vi "Close.vi"(8 "error in (no error)":errorcluster, 11 "State in":T1={"State"=enum."Idle", "Start Time"=timestamp(0 s since 1904-01-01), "Configuration"={"Cycle Period"=0.0, "PID 2 Parameters"={"Input Device"=enum."4-20mA", "Output Device"=enum."Default", "Setpoint"=0.0, "PID gains"={"proportional gain (Kc)"=0.0, "integral time (Ti, min)"=0.0, "derivative time (Td, min)"=100.0}, "output range"={"output low"=0.0, "output high"=1.0}}, "Manual Entry"=0.0, "Auto?"=TRUE, "4-20mA Input Settings"={"Input Channel "=0}, "4-20mA Out Settings"={"Output DAQ Task"=""}, "Input Channel Tag Name "=""}, "Current Time"=timestamp(0 s since 1904-01-01), "PID 1 Parameters"={"Setpoint"=0.0, "PID gains"={"proportional gain (Kc)"=1.0, "integral time (Ti, min)"=0.01, "derivative time (Td, min)"=0.0}}, "First Iteration"=FALSE, "Data"={"4-20mA Input"=0.0, "PID 2 Process Variable"=0.0, "PID 2 Output"=0.0, "4-20mA Output"=0.0}, "Process Name"="", "Pump On?"=enum."Off", "Input Error"=FALSE, "Output Error"=FALSE, "Log Started"=FALSE} {"Configuration"."PID 2 Parameters"."output range"."output low" format="%.2f"; "Configuration"."PID 2 Parameters"."output range"."output high" min=0.0 max=100.0 format="%.2f"; "Configuration"."PID 2 Parameters"."PID gains"."derivative time (Td, min)" format="%.3f"; "Configuration"."PID 2 Parameters"."PID gains"."integral time (Ti, min)" format="%.3f"; "Configuration"."PID 2 Parameters"."PID gains"."proportional gain (Kc)" format="%.3f"; "PID 1 Parameters"."PID gains"."derivative time (Td, min)" format="%.3f"; "PID 1 Parameters"."PID gains"."integral time (Ti, min)" format="%.3f"; "PID 1 Parameters"."PID gains"."proportional gain (Kc)" format="%.3f"}) -> (0 "error out":errorcluster, 3 "State out":T1={"State"=enum."Idle", "Start Time"=timestamp(0 s since 1904-01-01), "Configuration"={"Cycle Period"=0.0, "PID 2 Parameters"={"Input Device"=enum."4-20mA", "Output Device"=enum."Default", "Setpoint"=0.0, "PID gains"={"proportional gain (Kc)"=0.0, "integral time (Ti, min)"=0.0, "derivative time (Td, min)"=100.0}, "output range"={"output low"=0.0, "output high"=1.0}}, "Manual Entry"=0.0, "Auto?"=TRUE, "4-20mA Input Settings"={"Input Channel "=0}, "4-20mA Out Settings"={"Output DAQ Task"=""}, "Input Channel Tag Name "=""}, "Current Time"=timestamp(0 s since 1904-01-01), "PID 1 Parameters"={"Setpoint"=0.0, "PID gains"={"proportional gain (Kc)"=1.0, "integral time (Ti, min)"=0.01, "derivative time (Td, min)"=0.0}}, "First Iteration"=FALSE, "Data"={"4-20mA Input"=0.0, "PID 2 Process Variable"=0.0, "PID 2 Output"=0.0, "4-20mA Output"=0.0}, "Process Name"="", "Pump On?"=enum."Off", "Input Error"=FALSE, "Output Error"=FALSE, "Log Started"=FALSE} {"Configuration"."PID 2 Parameters"."output range"."output low" format="%.2f"; "Configuration"."PID 2 Parameters"."output range"."output high" min=0.0 max=100.0 format="%.2f"; "Configuration"."PID 2 Parameters"."PID gains"."derivative time (Td, min)" format="%.3f"; "Configuration"."PID 2 Parameters"."PID gains"."integral time (Ti, min)" format="%.3f"; "Configuration"."PID 2 Parameters"."PID gains"."proportional gain (Kc)" format="%.3f"; "PID 1 Parameters"."PID gains"."derivative time (Td, min)" format="%.3f"; "PID 1 Parameters"."PID gains"."integral time (Ti, min)" format="%.3f"; "PID 1 Parameters"."PID gains"."proportional gain (Kc)" format="%.3f"})   [LabVIEW 2018, in "4-20mA Module.lvlib" / "4-20mA Module Engine.lvlib"]
uses:
  4-20mA Module Engine.lvlib
  State Cluster.ctl
  State Enum.ctl
  Pressure Transmitter/Pressure Transmitter Device Settings.ctl
  Pressure Reg Module/Pressure Regulator Device Settings.ctl
  Measure Instrument/PID 1 Parameters Cluster.ctl
  Pressure Transmitter/Pressure Transmitter Library.lvlib
  Pressure Reg Module/Pressure Regulator Library.lvlib
panel:
  # "Instrument Settings"
  # "Instrument Settings"
  # "Instrument Settings"
  # "Instrument Settings"
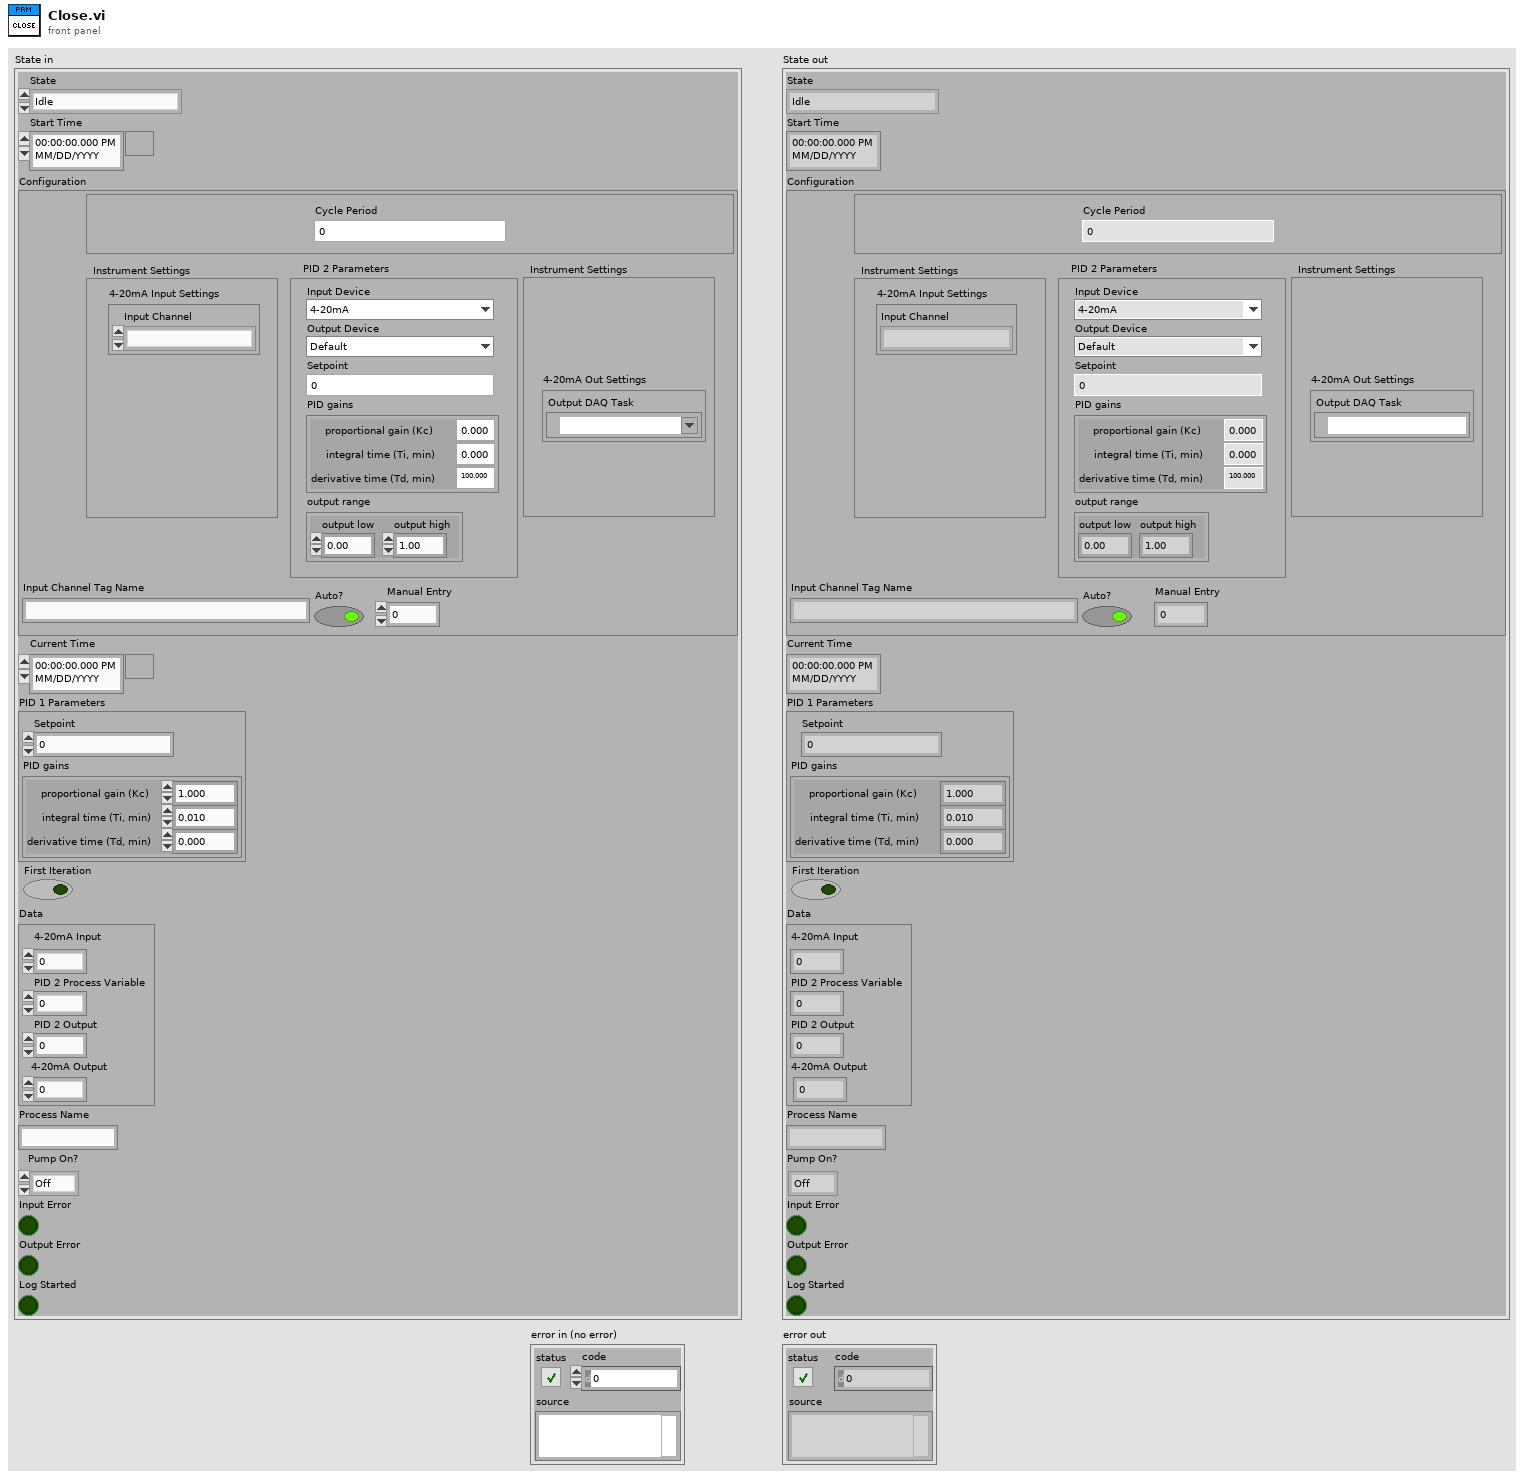
[diagram p1: front panel]
types:
  T1 = typedef "4-20mA Module.lvlib/4-20mA Module Engine.lvlib/State Cluster.ctl" = cluster{"State":T2, "Start Time":timestamp, "Configuration":cluster{"Cycle Period":dbl, "PID 2 Parameters":cluster{"Input Device":enum16{"Default", "4-20mA"}, "Output Device":enum16{"Default", "4-20mA"}, "Setpoint":dbl, "PID gains":cluster{"proportional gain (Kc)":dbl, "integral time (Ti, min)":dbl, "derivative time (Td, min)":dbl}, "output range":cluster{"output low":dbl, "output high":dbl}}, "Manual Entry":dbl, "Auto?":bool, "4-20mA Input Settings":T3, "4-20mA Out Settings":T4, "Input Channel Tag Name ":string}, "Current Time":timestamp, "PID 1 Parameters":T5, "First Iteration":bool, "Data":cluster{"4-20mA Input":dbl, "PID 2 Process Variable":dbl, "PID 2 Output":dbl, "4-20mA Output":dbl}, "Process Name":string, "Pump On?":enum16{"Off", "On", "Not Initialized"}, "Input Error":bool, "Output Error":bool, "Log Started":bool}
  T2 = typedef "4-20mA Module.lvlib/4-20mA Module Engine.lvlib/State Enum.ctl" = enum16{"Measuring", "Idle", "Paused"}
  T3 = typedef "Pressure Transmitter Library.lvlib/Pressure Transmitter Device Settings.ctl" = cluster{"Input Channel ":u16}
  T4 = typedef "Pressure Regulator Library.lvlib/Pressure Regulator Device Settings.ctl" = cluster{"Output DAQ Task":refnum<k21>}
  T5 = typedef "PID 1 Parameters Cluster.ctl" = cluster{"Setpoint":dbl, "PID gains":cluster{"proportional gain (Kc)":dbl, "integral time (Ti, min)":dbl, "derivative time (Td, min)":dbl}}
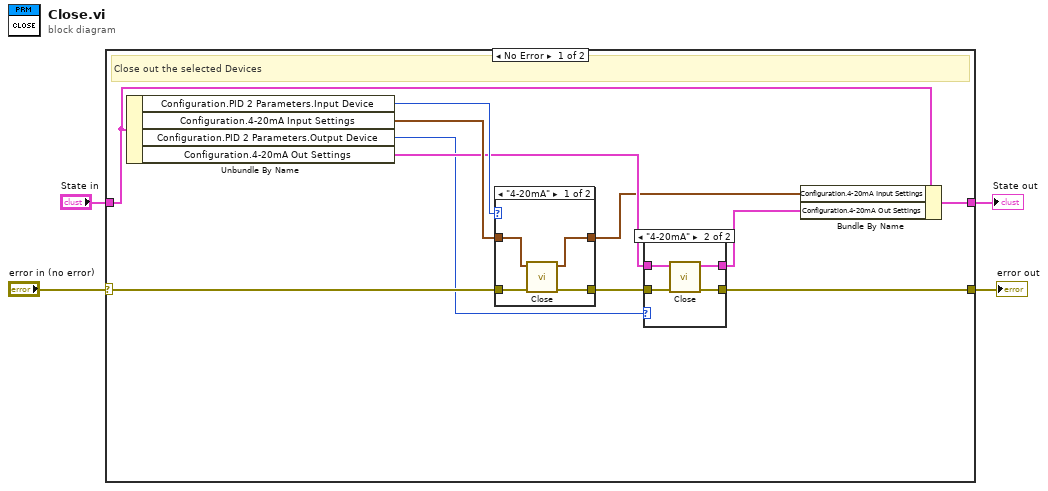
[diagram p0: block diagram]
diagram:
  n1 = case shown="No Error" "error in (no error)" {
    selector: "error in (no error)" -> [w13 w29]
    tunnel: [w10 w29] -> w3
    tunnel: "State in" -> [w7 w28]
    tunnel: [w12 w28] -> w2
    frame No Error {
      # "Close out the selected Devices"
      n2 = Unbundle By Name(w7) -> ("Configuration.PID 2 Parameters.Input Device"=w15:enum16{"Default", "4-20mA"}, "Configuration.4-20mA Input Settings"=w14:T3, "Configuration.PID 2 Parameters.Output Device"=w8:enum16{"Default", "4-20mA"}, "Configuration.4-20mA Out Settings"=w11:T4)
      n3 = case shown="\"4-20mA\"" w15 {
        tunnel: w14 -> [w22 w26]
        tunnel: w13 -> [w25 w27]
        tunnel: [w24 w27] -> w9
        tunnel: [w23 w26] -> w5
        frame "4-20mA" {
          n4 = call "Close.vi"("error in"=w25, "4-20mA Settings In"=w22) -> ("error out"=w24:errorcluster, "4-20mA Settings Out"=w23:T3)  [unwired: 8 in]
        }
        frame "Default", Default {
        }
      }
      n5 = case shown="\"4-20mA\"" w8 {
        tunnel: w11 -> [w16 w18]
        tunnel: [w17 w20] -> w10
        tunnel: w9 -> [w17 w21]
        tunnel: [w16 w19] -> w6
        frame "Default", Default {
        }
        frame "4-20mA" {
          n6 = call "Close.vi"("error in"=w21, "4-20mA Out Settings In"=w18) -> ("error out"=w20:errorcluster, "4-20mA Out Settings Out"=w19:T4)  [unwired: 8 in]
        }
      }
      n7 = Bundle By Name(cluster=w7, "Configuration.4-20mA Input Settings"=w5, "Configuration.4-20mA Out Settings"=w6) -> (w12:T1)
    }
    frame Error {
    }
  }
  "error out" <- w3
  "State out" <- w2
